vi "TimedPeakStreaming.vi"(6 "Number of peaks":i32, 7 "Number of channels":i32, 8 "Error In":errorcluster, 9 "Cycle period":dbl, 10 "Peaks buffer":dbl[][](array[numeric]), 11 "Address":string="10.0.0.55") -> (0 "Error Out":errorcluster, 1 "Peaks per channel":i32[](array[numeric]), 3 "Peaks":dbl[](array[numeric]))   [LabVIEW 2016]
doc: "This example VI demonstrates the establishment and use of streaming peaks data from Hyperion instruments."
uses:
  hyperion library source/h.Library/COMM/CTL/h.COMM.Socket Type.ctl
  hyperion library source/h.Library.lvlib
panel:
  out "Waveform Graph":dbl[][](graph)
  in  "Data Rate Divider":i32=1 min=1 step=1
  # "Hyperion Timed Streaming"
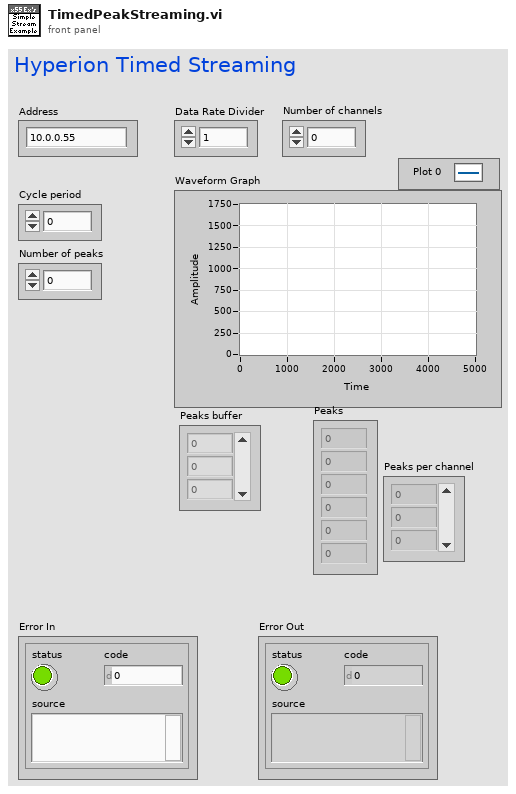
[diagram p1: front panel]
types:
  T1 = typedef "h.Library.lvlib/h.COMM.Socket Type.ctl" = u16
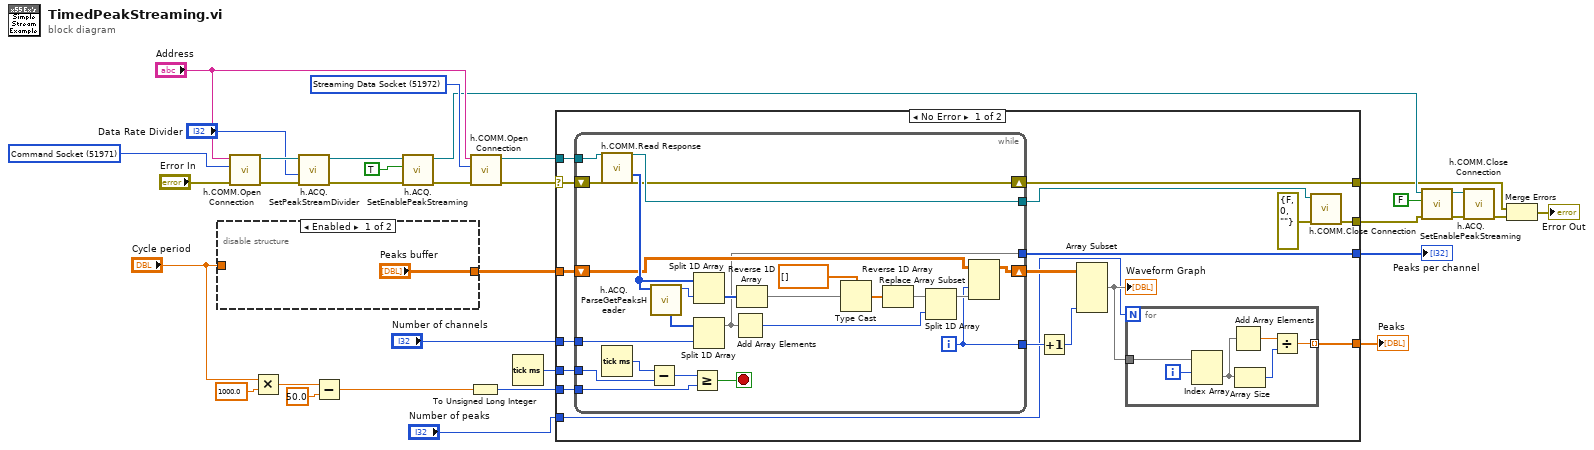
[diagram p0: block diagram]
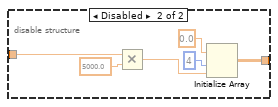
[diagram p2: hidden frame]
diagram:
  w26 = T1 51972 items=["Command Socket"=51971, "Streaming Data Socket"=51972] ("Port")
  w27 = T1 51971 items=["Command Socket"=51971, "Streaming Data Socket"=51972] ("Port")
  n1 = disable-structure shown="Enabled" {
    disable-tunnel: ["Peaks buffer" w37] -> w6
    disable-tunnel: "Cycle period" -> [_ w38]
    frame Enabled {
    }
    frame Disabled {
      n2 = Multiply(x=w38, y=5000.0) -> (x*y=w35:dbl)
      n3 = Initialize Array(0.0, 4 ("dimension size"), w35) -> (w37:dbl[][])
    }
  }
  n4 = call "h.COMM.Open Connection.vi"("error in"="Error In", "Port"=w27, "Address"="Address") -> ("error out"=w31:errorcluster, "Connection ID"=w33:refnum<k5>)  [unwired: 7 in]
  n5 = Multiply(x="Cycle period", y=1000.0) -> (x*y=w14:dbl)
  n6 = call "h.ACQ.SetPeakStreamDivider.vi"("error in"=w31, "Data Rate Divider"="Data Rate Divider", "Connection ID In"=w33) -> ("error out"=w23:errorcluster, "Connection ID Out"=w25:refnum<k5>)  [unwired: 7 in]
  n7 = Subtract(x=w14, y=50.0) -> (x-y=w12:dbl)
  n8 = call "h.ACQ.SetEnablePeakStreaming.vi"("error in"=w23, "Enable"=TRUE, "Connection ID in"=w25) -> ("error out"=w22:errorcluster, "Connection ID out"=w19:refnum<k5>)  [unwired: 7 in]
  n9 = To Unsigned Long Integer(number=w12) -> (unsigned 32bit integer=w10:u32)
  n10 = call "h.COMM.Open Connection.vi"("error in"=w22, "Port"=w26, "Address"="Address") -> ("error out"=w29:errorcluster, "Connection ID"=w28:refnum<k5>)  [unwired: 7 in]
  n11 = Tick Count (ms)() -> (millisecond timer value=w11:u32)
  n12 = case shown="No Error" w29 {
    selector: w29 -> [w56 w88]
    tunnel: w28 -> [w54 _]
    tunnel: [w53 _] -> w20
    tunnel: w11 -> [w52 _]
    tunnel: w10 -> [w51 _]
    tunnel: [w50 w88] -> w9
    tunnel: w6 -> [w49 _]
    tunnel: [w47 _] -> w4
    tunnel: "Number of peaks" -> [w43 _]
    tunnel: "Number of channels" -> [w42 _]
    tunnel: [w41 _] -> w1
    frame No Error {
      n13 = while {
        tunnel: [w71] -> w57
        shift-right: [w69] -> w50
        shift-left: w56 -> [w70]
        tunnel: w54 -> [w82]
        tunnel: w52 -> [w86]
        tunnel: w51 -> [w84]
        shift-right: [w72] -> w48
        shift-left: w49 -> [w74]
        tunnel: [w68] -> w46
        tunnel: w42 -> [w66]
        tunnel: [w64] -> w41
        i -> [w68]
        stop <- w83 stop-if-true
        n14 = call "h.COMM.Read Response.vi"("Connection ID"=w82, "error in"=w70) -> ("Connection ID"=w71:refnum<k5>, "Content"=w81:u8[], "error out"=w69:errorcluster)  [unwired: 18 in, 5 out]
        n15 = Tick Count (ms)() -> (millisecond timer value=w87:u32)
        n16 = Subtract(x=w87, y=w86) -> (x-y=w85:u32)
        n17 = call "h.ACQ.ParseGetPeaksHeader.vi"("Header from #GetPeaks"=w81) -> ("Header Length"=w80:u16, "#Peaks"=w67:u16[])  [unwired: 6 in, 3 out]
        n18 = Greater Or Equal?(x=w85, y=w84) -> (x >= y?=w83:bool)
        n19 = Split 1D Array(array=w81, index=w80) -> (second subarray=w79:u8[])  [unwired: 1 out]
        n20 = Split 1D Array(array=w67, index=w66) -> (first subarray=w64:u16[])  [unwired: 1 out]
        n21 = Add Array Elements(numeric array=w64) -> (sum=w65:u16)
        n22 = Reverse 1D Array(array=w79) -> (reversed array=w76:u8[])
        n23 = Type Cast(type=dbl[] [], x=w76) -> (*(type *) &x=w78:dbl[])
        n24 = Reverse 1D Array(array=w78) -> (reversed array=w75:dbl[])
        n25 = Split 1D Array(array=w75, index=w65) -> (first subarray=w73:dbl[])  [unwired: 1 out]
        n26 = Replace Array Subset(array=w74, new element=w73, index (col)=w68) -> (w72:dbl[][])  [unwired: 1 in]
      }
      n27 = Increment(x=w46) -> (x+1=w44:i32)
      n28 = Array Subset(array=w48, length (col)=w44) -> (w45:dbl[][])  [unwired: 3 in]
      "Waveform Graph" <- w45
      n29 = for {
        N: w43 -> [_]
        tunnel: w45 -> [w63]
        tunnel: [w59] -> w47 mode=indexing
        i -> [w58]
        n30 = Index Array(array=w63, index (row)=w58) -> (element=w62:dbl[])  [unwired: 1 in]
        n31 = Add Array Elements(numeric array=w62) -> (sum=w61:dbl)
        n32 = Array Size(array=w62) -> (size(s)=w60:i32)
        n33 = Divide(x=w61, y=w60) -> (x/y=w59:dbl)
      }
      n34 = call "h.COMM.Close Connection.vi"("error in"=errorcluster {"status"=FALSE, "code"=0, "source"=""}, "Connection ID"=w57) -> ("error out"=w53:errorcluster)  [unwired: 9 in]
    }
    frame Error {
    }
  }
  "Peaks" <- w4
  "Peaks per channel" <- w1
  n35 = call "h.ACQ.SetEnablePeakStreaming.vi"("error in"=w20, "Enable"=FALSE, "Connection ID in"=w19) -> ("error out"=w18:errorcluster, "Connection ID out"=w17:refnum<k5>)  [unwired: 7 in]
  n36 = call "h.COMM.Close Connection.vi"("error in"=w18, "Connection ID"=w17) -> ("error out"=w7:errorcluster)  [unwired: 9 in]
  n37 = Merge Errors(w9, w7) -> (→"Error Out":errorcluster)
